vi "Split-Input-Stream.vi"(11 "Raw Data\nStream":u64[](array[numeric])=[68719476735, 68719411202, 67802302532, 64559120385, 64558728708, 64424574978, 67802302532, 64592281956, 64424509440, 64424512000, 64447905792, 64424509440, 64424509440, 64424509440, 64424509440, 66519609314, 281539401220098, 68719476735, 68719411202, 67802302532, 64559120385, 64558728708, 64424574978, 67802302532, 64592281956, 64424509440, 64424512000, 64447905792, 64424509440, 64424509440, 64424509440, 64424509440, 66519609314, 281539401220098, 68719476735, 68719411202, 67802302532, 64559120385, 64558728708, 64424574978, 67802302532, 64592281956, 64424509440, 64424512000, 64447905792, 64424509440, 64424509440, 64424509440, 64424509440, 66519609314, 281539401220098] format="%.0x") -> (3 "Array":u32[][](array[numeric]) format="%.0x")   [LabVIEW 2018]
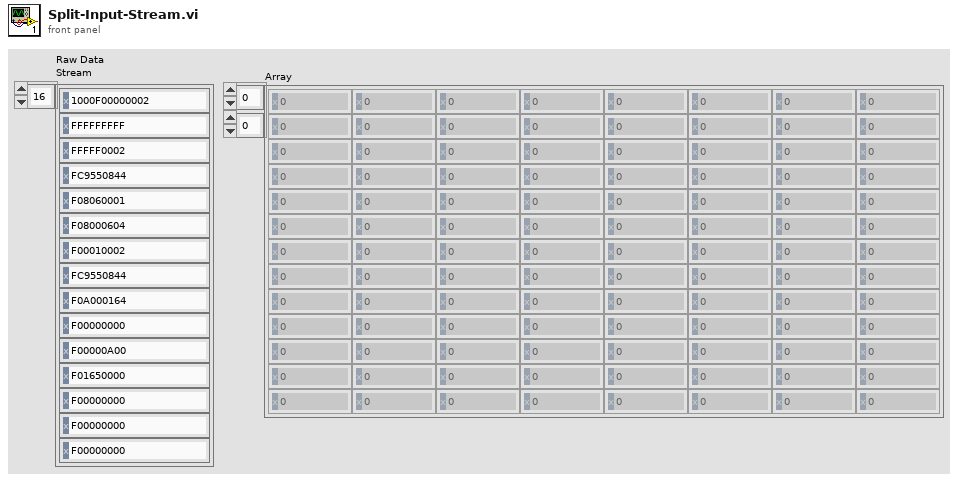
[diagram p1: front panel]
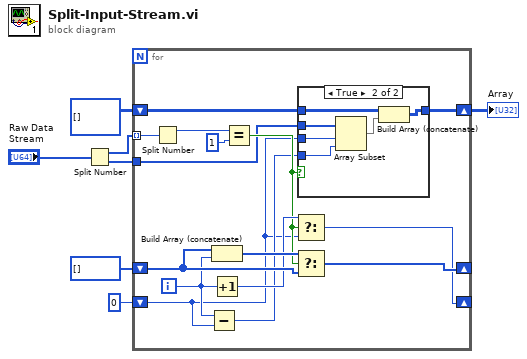
[diagram p0: block diagram]
diagram:
  n1 = Split Number(x="Raw Data\nStream") -> (hi(x)=w3:u32[], lo(x)=w1:u32[])
  n2 = for {
    tunnel: w3 -> [w22] mode=indexing
    shift-right: [w19] -> _
    shift-left: u16[] [] -> [w17]
    shift-right: [w14] -> _
    shift-left: 0 -> [w8]
    shift-right: [w9] -> w4
    shift-left: u32[][] [] -> [w10]
    tunnel: w1 -> [w12]
    i -> [w15]
    n3 = Split Number(x=w22) -> (hi(x)=w21:u16)  [unwired: 1 out]
    n4 = Subtract(x=w15, y=w8) -> (x-y=w11:i32)
    n5 = Build Array (concatenate)(w17, w15) -> (w18:i32[])
    n6 = Increment(x=w15) -> (x+1=w16:i32)
    n7 = Equal?(x=w21, y=u16 1) -> (x = y?=w13:bool)
    n8 = Select(t=w16, s=w13, f=w8) -> (s? t:f=w14:i32)
    n9 = Select(t=w18, s=w13, f=w17) -> (s? t:f=w19:i32[])
    n10 = case shown="True" w13 {
      tunnel: w12 -> [_ w29]
      tunnel: w8 -> [_ w28]
      tunnel: w11 -> [_ w27]
      tunnel: w10 -> [w23 w26]
      tunnel: [w23 w25] -> w9
      frame False {
      }
      frame True {
        n11 = Array Subset(array=w29, index=w28, length=w27) -> (w24:u32[])
        n12 = Build Array (concatenate)(w26, w24) -> (w25:u32[][])
      }
    }
  }
  "Array" <- w4
